vi "disable-structure-frame-names.vi"   [LabVIEW 2025]
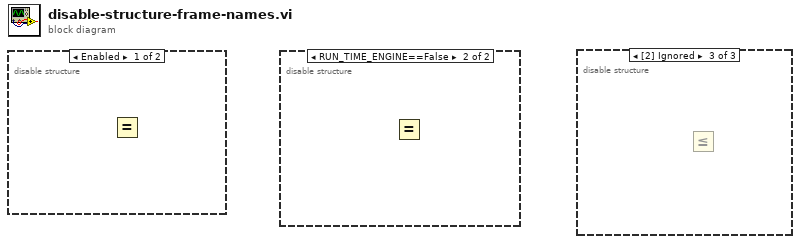
[diagram p0: block diagram]
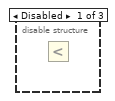
[diagram p2: hidden frame]
diagram:
  n1 = disable-structure "Diagram Disable Structure" shown="Enabled" {
    frame Enabled {
      n2 = Equal?() -> ()  [unwired: 2 in, 1 out]
    }
    frame Disabled {
    }
  }
  n3 = disable-structure "Conditional Disable Structure" shown="RUN_TIME_ENGINE==False" {
    frame condition #0 {
    }
    frame condition #1 (active) {
      n4 = Equal?() -> ()  [unwired: 2 in, 1 out]
    }
  }
  n5 = disable-structure "Type Specialization Structure" shown="[2] Ignored" {
    frame Disabled {
      n6 = Less?() -> ()  [unwired: 2 in, 1 out]
    }
    frame Enabled {
    }
    frame Disabled {
      n7 = Less Or Equal?() -> ()  [unwired: 2 in, 1 out]
    }
  }
